vi "PRIME Gen Filenames and Log.vi"(9 "Observation":T1={"Priority"=0, "ID"="", "Observer"="", "Obj Name"="", "Obj Type"="", "RA and DEC String"={"RA"="HH:MM:SS.nnn", "DEC"="DEG:arcmin:arcsec.nn"}, "Filters"=[], "Integration Time"=0.0, "Observation Status"=enum."Error", "Offsets"={"RA"=0.0, "DEC"=0.0, "ROT"=0.0}, "Images"=0, "Dither Options"={"Dither"=enum."None", "Dither Radius"=0.0, "Dither Points"=0, "Dither Phase"=0.0, "B Offset"={"RA"=0.0, "DEC"=0.0}}, "Comment 1"="", "Comment 2"=""}, 10 "Detector Config":T8={"Detector"=0, "Offsets"=[[0, 0, 0, 0, 0, 0, 0, 0, 0, 0, 0, 0, 0, 0, 0, 0, 0, 0, 0, 0, 0, 0, 0, 0, 0, 0, 0, 0, 0, 0, 0, 0]], "Detector Computer"={"Machine"="192.168.121.11", "Password"="rSL!nux23456", "FITS File Path"="", "Port"=44444, "Header Path"="", "Name"=""}, "FITS hdr template0"=path "", "FITS hdr template1"=path "", "FITS Data File Path"=path "", "FITS Detector Settings"={"Exp Time Short"=0.0, "# of Frames"=0.0, "Exp Time Long"=0.0, "# of Groups"=0.0, "Object Name"="", "Object"="", "Obs Type"="", "Image Type"="", "Observer"="", "Observer Affiliation"=""}, "Sim Folder"=path "", "Integration Mode"=enum."Ramp", "Integration Time"=0.0, "Frame Int Time"=0.0} {"Offsets" format="%04x"; "Detector" items=["0", "1", "2"]}, 11 "Raw Files":T7) -> (0 "Exp Count out":i32, 1 "Source Files":path[](array[path]), 2 "Filenames":string[](array[string]), 3 "Table":string[](array[string]))   [LabVIEW 2024, in "PRIME Detector.lvclass"]
uses:
  PRIME Detector.lvclass
  RIMAS Detector Config.ctl
  RIMAS Detector Server Config.ctl
  RIMAS Observation Config.ctl
  Detector enum Detector Integration Mode.ctl
  Detector cluster Files.ctl
  typedefs/CC cluster Observation.ctl
  Observation Queue/CC enum Observation Status.ctl
  Telescope/CC cluster Telescope Offsets.ctl
  typedefs/CC cluster Observation Dither Options.ctl
  typedefs/CC enum Dither Selection.ctl
  typedefs/CC cluster RA and DEC.ctl
  PRIME Detector cluster Status.ctl
  FITS/PRIME cluster File Counter.ctl
  Logging/CC enum Current Values Action.ctl
  hk-channel-class/hk-channel-class/HK Table/HK Table.lvclass
  Detector Class.lvclass
panel:
  # "sec"
  # "sec"
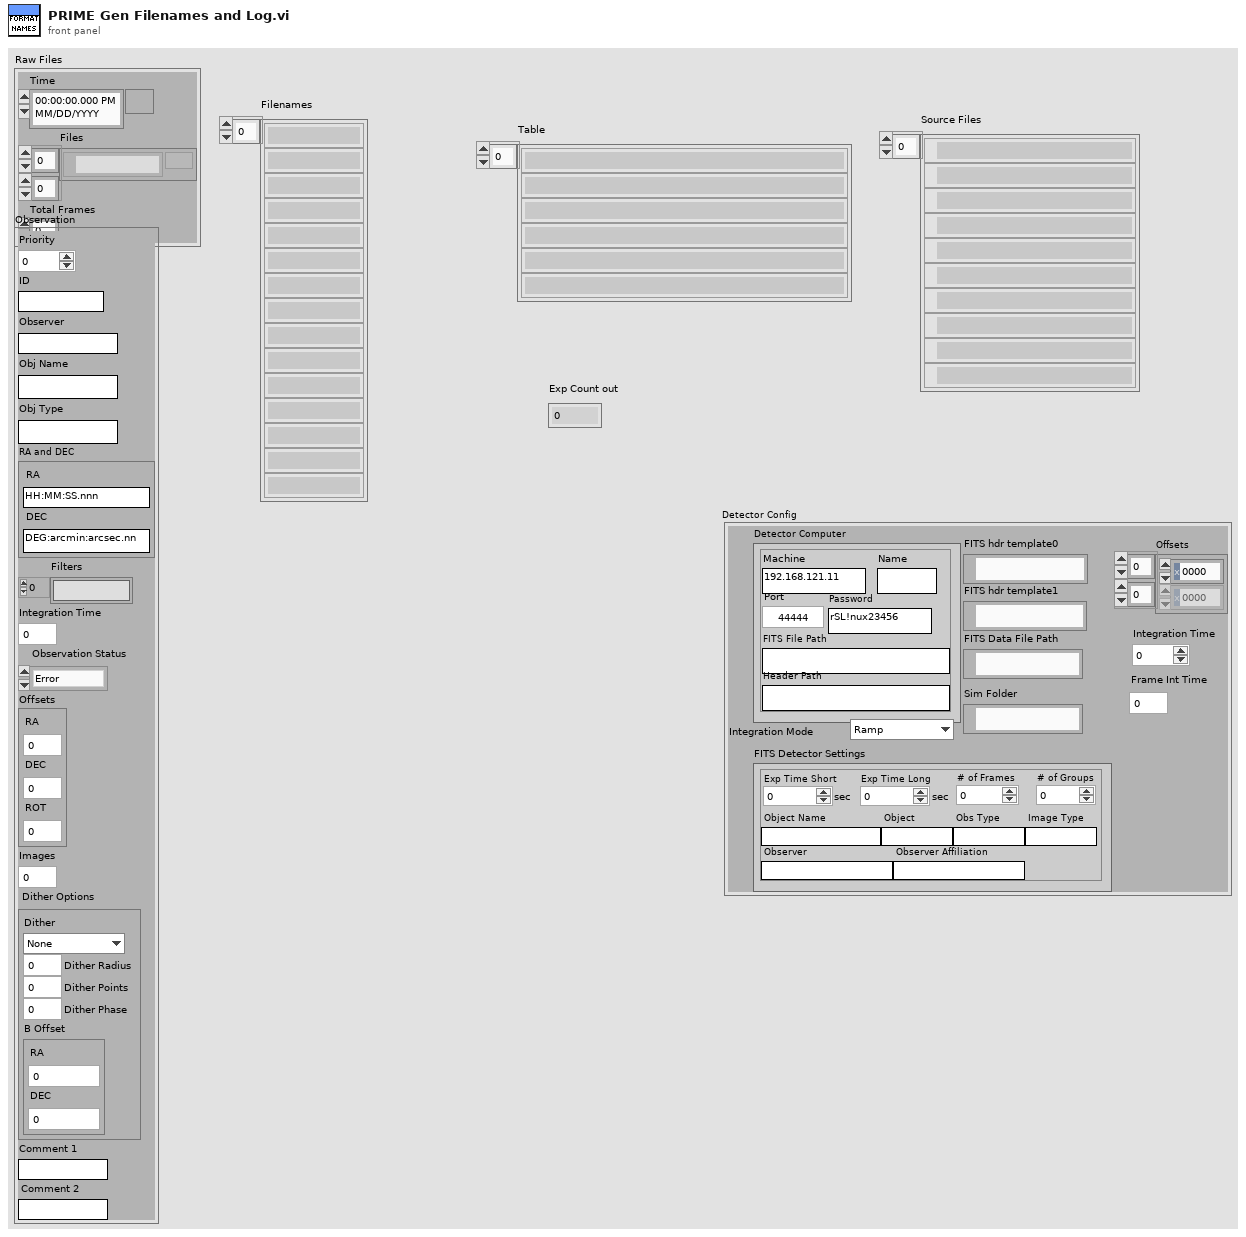
[diagram p1: front panel]
types:
  T1 = typedef "CC cluster Observation.ctl" = cluster{"Priority":i32, "ID":string, "Observer":string, "Obj Name":string, "Obj Type":string, "RA and DEC String":cluster{"RA":string, "DEC":string}, "Filters":string[], "Integration Time":dbl, "Observation Status":T2, "Offsets":T3, "Images":i32, "Dither Options":T4, "Comment 1":string, "Comment 2":string}
  T2 = typedef "CC enum Observation Status.ctl" = enum16{"Ready", "Running", "Done", "Error"}
  T3 = typedef "CC cluster Telescope Offsets.ctl" = cluster{"RA":dbl, "DEC":dbl, "ROT":dbl}
  T4 = typedef "CC cluster Observation Dither Options.ctl" = cluster{"Dither":T5, "Dither Radius":dbl, "Dither Points":i32, "Dither Phase":dbl, "B Offset":T6}
  T5 = typedef "CC enum Dither Selection.ctl" = enum16{"None", "Circle", "Random", "ABBA"}
  T6 = typedef "CC cluster RA and DEC.ctl" = cluster{"RA":dbl, "DEC":dbl}
  T7 = typedef "Detector Class.lvclass/Detector cluster Files.ctl" = cluster{"Time":timestamp, "Files":path[][], "Total Frames":i32}
  T8 = typedef "RIMAS Detector Config.ctl" = cluster{"Detector":u16, "Offsets":u16[][], "Detector Computer":T9, "FITS hdr template0":path, "FITS hdr template1":path, "FITS Data File Path":path, "FITS Detector Settings":T10, "Sim Folder":path, "Integration Mode":T11, "Integration Time":dbl, "Frame Int Time":dbl}
  T9 = typedef "RIMAS Detector Server Config.ctl" = cluster{"Machine":string, "Password":string, "FITS File Path":string, "Port":u16, "Header Path":string, "Name":string}
  T10 = typedef "RIMAS Observation Config.ctl" = cluster{"Exp Time Short":dbl, "# of Frames":dbl, "Exp Time Long":dbl, "# of Groups":dbl, "Object Name":string, "Object":string, "Obs Type":string, "Image Type":string, "Observer":string, "Observer Affiliation":string}
  T11 = typedef "Detector enum Detector Integration Mode.ctl" = enum16{"Ramp", "CDS", "FOWLER2", "FOWLER4", "FOWLER8", "FOWLER16", "Raw"}
  T12 = typedef "CC enum Current Values Action.ctl" = enum16{"Init", "Write Item", "Write Array", "Read Item", "Read Array", "Read All", "Add Channels", "New File", "Add Message", "Get Current Values", "Close"}
  T13 = typedef "PRIME cluster File Counter.ctl" = cluster{"File Count":i32}
  T14 = typedef "PRIME Detector cluster Status.ctl" = cluster{"Cmd Start Time":timestamp, "Command":string, "Complete?":bool, "Cmd Complete Time":timestamp, "Exp Time Remaining":dbl, "Total Frames":i32, "Exp Frames":cluster{"CAMERA0":string[], "CAMERA1":string[], "CAMERA2":string[], "CAMERA3":string[]}, "Intermediate Frames":cluster{"CAMERA0":string[], "CAMERA1":string[], "CAMERA2":string[], "CAMERA3":string[]}, "Final Reduced Frame":cluster{"CAMERA0":string, "CAMERA1":string, "CAMERA2":string, "CAMERA3":string}}
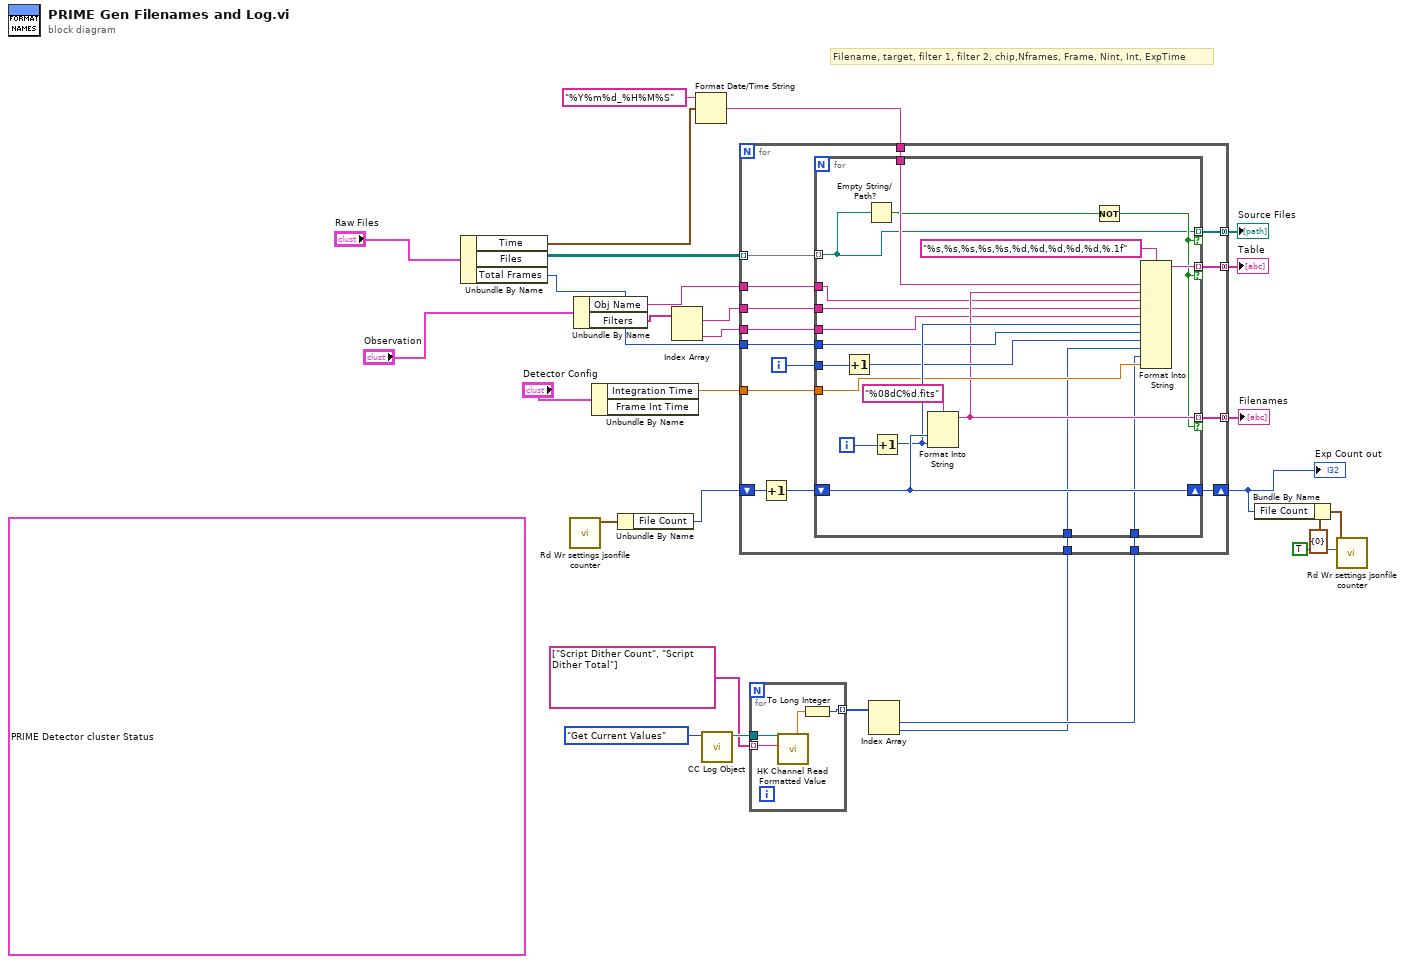
[diagram p0: block diagram]
diagram:
  (unwired) T14 {"Cmd Start Time"=timestamp(3729599083.065959 s since 1904-01-01), "Command"="START", "Complete?"=TRUE, "Cmd Complete Time"=timestamp(3729599162.21691 s since 1904-01-01), "Exp Time Remaining"=0.0, "Total Frames"=8, "Exp Frames"={"CAMERA0"=["C:\\Users\\gsfcprime\\PycharmProjects\\asdetector\\output\\raw\\20220308\\prime.0000.C0\\prime.0000.C0.000000.fits", "C:\\Users\\gsfcprime\\PycharmProjects\\asdetector\\output\\raw\\20220308\\prime.0000.C0\\prime.0000.C0.000001.fits", "C:\\Users\\gsfcprime\\PycharmProjects\\asdetector\\output\\raw\\20220308\\prime.0000.C0\\prime.0000.C0.000002.fits", "C:\\Users\\gsfcprime\\PycharmProjects\\asdetector\\output\\raw\\20220308\\prime.0000.C0\\prime.0000.C0.000003.fits", "C:\\Users\\gsfcprime\\PycharmProjects\\asdetector\\output\\raw\\20220308\\prime.0000.C0\\prime.0000.C0.000004.fits", "C:\\Users\\gsfcprime\\PycharmProjects\\asdetector\\output\\raw\\20220308\\prime.0000.C0\\prime.0000.C0.000005.fits", "C:\\Users\\gsfcprime\\PycharmProjects\\asdetector\\output\\raw\\20220308\\prime.0000.C0\\prime.0000.C0.000006.fits", "C:\\Users\\gsfcprime\\PycharmProjects\\asdetector\\output\\raw\\20220308\\prime.0000.C0\\prime.0000.C0.000007.fits"], "CAMERA1"=["C:\\Users\\gsfcprime\\PycharmProjects\\asdetector\\output\\raw\\20220308\\prime.0000.C1\\prime.0000.C1.000000.fits", "C:\\Users\\gsfcprime\\PycharmProjects\\asdetector\\output\\raw\\20220308\\prime.0000.C1\\prime.0000.C1.000001.fits", "C:\\Users\\gsfcprime\\PycharmProjects\\asdetector\\output\\raw\\20220308\\prime.0000.C1\\prime.0000.C1.000002.fits", "C:\\Users\\gsfcprime\\PycharmProjects\\asdetector\\output\\raw\\20220308\\prime.0000.C1\\prime.0000.C1.000003.fits", "C:\\Users\\gsfcprime\\PycharmProjects\\asdetector\\output\\raw\\20220308\\prime.0000.C1\\prime.0000.C1.000004.fits", "C:\\Users\\gsfcprime\\PycharmProjects\\asdetector\\output\\raw\\20220308\\prime.0000.C1\\prime.0000.C1.000005.fits", "C:\\Users\\gsfcprime\\PycharmProjects\\asdetector\\output\\raw\\20220308\\prime.0000.C1\\prime.0000.C1.000006.fits", "C:\\Users\\gsfcprime\\PycharmProjects\\asdetector\\output\\raw\\20220308\\prime.0000.C1\\prime.0000.C1.000007.fits"], "CAMERA2"=["C:\\Users\\gsfcprime\\PycharmProjects\\asdetector\\output\\raw\\20220308\\prime.0000.C2\\prime.0000.C2.000000.fits", "C:\\Users\\gsfcprime\\PycharmProjects\\asdetector\\output\\raw\\20220308\\prime.0000.C2\\prime.0000.C2.000001.fits", "C:\\Users\\gsfcprime\\PycharmProjects\\asdetector\\output\\raw\\20220308\\prime.0000.C2\\prime.0000.C2.000002.fits", "C:\\Users\\gsfcprime\\PycharmProjects\\asdetector\\output\\raw\\20220308\\prime.0000.C2\\prime.0000.C2.000003.fits", "C:\\Users\\gsfcprime\\PycharmProjects\\asdetector\\output\\raw\\20220308\\prime.0000.C2\\prime.0000.C2.000004.fits", "C:\\Users\\gsfcprime\\PycharmProjects\\asdetector\\output\\raw\\20220308\\prime.0000.C2\\prime.0000.C2.000005.fits", "C:\\Users\\gsfcprime\\PycharmProjects\\asdetector\\output\\raw\\20220308\\prime.0000.C2\\prime.0000.C2.000006.fits", "C:\\Users\\gsfcprime\\PycharmProjects\\asdetector\\output\\raw\\20220308\\prime.0000.C2\\prime.0000.C2.000007.fits"], "CAMERA3"=["C:\\Users\\gsfcprime\\PycharmProjects\\asdetector\\output\\raw\\20220308\\prime.0000.C3\\prime.0000.C3.000000.fits", "C:\\Users\\gsfcprime\\PycharmProjects\\asdetector\\output\\raw\\20220308\\prime.0000.C3\\prime.0000.C3.000001.fits", "C:\\Users\\gsfcprime\\PycharmProjects\\asdetector\\output\\raw\\20220308\\prime.0000.C3\\prime.0000.C3.000002.fits", "C:\\Users\\gsfcprime\\PycharmProjects\\asdetector\\output\\raw\\20220308\\prime.0000.C3\\prime.0000.C3.000003.fits", "C:\\Users\\gsfcprime\\PycharmProjects\\asdetector\\output\\raw\\20220308\\prime.0000.C3\\prime.0000.C3.000004.fits", "C:\\Users\\gsfcprime\\PycharmProjects\\asdetector\\output\\raw\\20220308\\prime.0000.C3\\prime.0000.C3.000005.fits", "C:\\Users\\gsfcprime\\PycharmProjects\\asdetector\\output\\raw\\20220308\\prime.0000.C3\\prime.0000.C3.000006.fits", "C:\\Users\\gsfcprime\\PycharmProjects\\asdetector\\output\\raw\\20220308\\prime.0000.C3\\prime.0000.C3.000007.fits"]}, "Intermediate Frames"={"CAMERA0"=["C:\\Users\\gsfcprime\\PycharmProjects\\asdetector\\output\\res\\20220308\\prime.0000.C0\\prime.0000.C0.000000.fits", "C:\\Users\\gsfcprime\\PycharmProjects\\asdetector\\output\\res\\20220308\\prime.0000.C0\\prime.0000.C0.000001.fits", "C:\\Users\\gsfcprime\\PycharmProjects\\asdetector\\output\\res\\20220308\\prime.0000.C0\\prime.0000.C0.000002.fits", "C:\\Users\\gsfcprime\\PycharmProjects\\asdetector\\output\\res\\20220308\\prime.0000.C0\\prime.0000.C0.000003.fits", "C:\\Users\\gsfcprime\\PycharmProjects\\asdetector\\output\\res\\20220308\\prime.0000.C0\\prime.0000.C0.000004.fits", "C:\\Users\\gsfcprime\\PycharmProjects\\asdetector\\output\\res\\20220308\\prime.0000.C0\\prime.0000.C0.000005.fits", "C:\\Users\\gsfcprime\\PycharmProjects\\asdetector\\output\\res\\20220308\\prime.0000.C0\\prime.0000.C0.000006.fits", "C:\\Users\\gsfcprime\\PycharmProjects\\asdetector\\output\\res\\20220308\\prime.0000.C0\\prime.0000.C0.000007.fits"], "CAMERA1"=["C:\\Users\\gsfcprime\\PycharmProjects\\asdetector\\output\\res\\20220308\\prime.0000.C1\\prime.0000.C1.000000.fits", "C:\\Users\\gsfcprime\\PycharmProjects\\asdetector\\output\\res\\20220308\\prime.0000.C1\\prime.0000.C1.000001.fits", "C:\\Users\\gsfcprime\\PycharmProjects\\asdetector\\output\\res\\20220308\\prime.0000.C1\\prime.0000.C1.000002.fits", "C:\\Users\\gsfcprime\\PycharmProjects\\asdetector\\output\\res\\20220308\\prime.0000.C1\\prime.0000.C1.000003.fits", "C:\\Users\\gsfcprime\\PycharmProjects\\asdetector\\output\\res\\20220308\\prime.0000.C1\\prime.0000.C1.000004.fits", "C:\\Users\\gsfcprime\\PycharmProjects\\asdetector\\output\\res\\20220308\\prime.0000.C1\\prime.0000.C1.000005.fits", "C:\\Users\\gsfcprime\\PycharmProjects\\asdetector\\output\\res\\20220308\\prime.0000.C1\\prime.0000.C1.000006.fits", "C:\\Users\\gsfcprime\\PycharmProjects\\asdetector\\output\\res\\20220308\\prime.0000.C1\\prime.0000.C1.000007.fits"], "CAMERA2"=["C:\\Users\\gsfcprime\\PycharmProjects\\asdetector\\output\\res\\20220308\\prime.0000.C2\\prime.0000.C2.000000.fits", "C:\\Users\\gsfcprime\\PycharmProjects\\asdetector\\output\\res\\20220308\\prime.0000.C2\\prime.0000.C2.000001.fits", "C:\\Users\\gsfcprime\\PycharmProjects\\asdetector\\output\\res\\20220308\\prime.0000.C2\\prime.0000.C2.000002.fits", "C:\\Users\\gsfcprime\\PycharmProjects\\asdetector\\output\\res\\20220308\\prime.0000.C2\\prime.0000.C2.000003.fits", "C:\\Users\\gsfcprime\\PycharmProjects\\asdetector\\output\\res\\20220308\\prime.0000.C2\\prime.0000.C2.000004.fits", "C:\\Users\\gsfcprime\\PycharmProjects\\asdetector\\output\\res\\20220308\\prime.0000.C2\\prime.0000.C2.000005.fits", "C:\\Users\\gsfcprime\\PycharmProjects\\asdetector\\output\\res\\20220308\\prime.0000.C2\\prime.0000.C2.000006.fits", "C:\\Users\\gsfcprime\\PycharmProjects\\asdetector\\output\\res\\20220308\\prime.0000.C2\\prime.0000.C2.000007.fits"], "CAMERA3"=["C:\\Users\\gsfcprime\\PycharmProjects\\asdetector\\output\\res\\20220308\\prime.0000.C3\\prime.0000.C3.000000.fits", "C:\\Users\\gsfcprime\\PycharmProjects\\asdetector\\output\\res\\20220308\\prime.0000.C3\\prime.0000.C3.000001.fits", "C:\\Users\\gsfcprime\\PycharmProjects\\asdetector\\output\\res\\20220308\\prime.0000.C3\\prime.0000.C3.000002.fits", "C:\\Users\\gsfcprime\\PycharmProjects\\asdetector\\output\\res\\20220308\\prime.0000.C3\\prime.0000.C3.000003.fits", "C:\\Users\\gsfcprime\\PycharmProjects\\asdetector\\output\\res\\20220308\\prime.0000.C3\\prime.0000.C3.000004.fits", "C:\\Users\\gsfcprime\\PycharmProjects\\asdetector\\output\\res\\20220308\\prime.0000.C3\\prime.0000.C3.000005.fits", "C:\\Users\\gsfcprime\\PycharmProjects\\asdetector\\output\\res\\20220308\\prime.0000.C3\\prime.0000.C3.000006.fits", "C:\\Users\\gsfcprime\\PycharmProjects\\asdetector\\output\\res\\20220308\\prime.0000.C3\\prime.0000.C3.000007.fits"]}, "Final Reduced Frame"={"CAMERA0"="C:\\Users\\gsfcprime\\PycharmProjects\\asdetector\\output\\reduced\\20220308\\prime.0000.C0.fits", "CAMERA1"="C:\\Users\\gsfcprime\\PycharmProjects\\asdetector\\output\\reduced\\20220308\\prime.0000.C1.fits", "CAMERA2"="C:\\Users\\gsfcprime\\PycharmProjects\\asdetector\\output\\reduced\\20220308\\prime.0000.C2.fits", "CAMERA3"="C:\\Users\\gsfcprime\\PycharmProjects\\asdetector\\output\\reduced\\20220308\\prime.0000.C3.fits"}} ("prime detector status")
  # "Filename, target, filter 1, filter 2, chip,Nframes, Frame, Nint, Int, ExpTime"
  n1 = Unbundle By Name("Raw Files") -> ("Time"=w8:timestamp, "Files"=w7:path[][], "Total Frames"=w6:i32)
  n2 = call "Rd Wr settings jsonfile counter.vi"() -> ("FileCounter"=w21:T13)  [unwired: 10 in, 1 out]
  n3 = Unbundle By Name("Observation") -> ("Obj Name"=w3:string, "Filters"=w4:string[])
  n4 = Unbundle By Name("Detector Config") -> ("Integration Time"=w26:dbl)  [unwired: 1 out]
  n5 = Unbundle By Name(w21) -> ("File Count"=w20:i32)
  n6 = Index Array(array=w4) -> (element #1=w2:string, element #2=w1:string)  [unwired: 2 in]
  n7 = Format Date/Time String(time format string (%c)="%Y%m%d_%H%M%S", seconds (now)=w8) -> (date/time string=w22:string)  [unwired: 1 in]
  n8 = call "CC Log Object.vi"("Action"=CC_enum_Current_Values_Action."Get Current Values") -> ("HK Channel out"=w14:refnum<class "HK Table.lvclass">)  [unwired: 8 in, 2 out]
  n9 = for {
    tunnel: w14 -> [w32]
    tunnel: string[] ["Script Dither Count", "Script Dither Total"] -> [w31] mode=indexing
    tunnel: [w29] -> w12 mode=indexing
    n10 = call-dynamic "HK Channel Read Formatted Value.vi"("Name"=w31, "HK Table.lvclass"=w32) -> ("Value"=w30:dbl)  [unwired: 2 in, 7 out]
    n11 = To Long Integer(number=w30) -> (32bit integer=w29:i32)
  }
  n12 = Index Array(array=w12) -> (element #1=w11:i32, element #2=w10:i32)  [unwired: 2 in]
  n13 = for {
    shift-right: [w48] -> w18
    shift-left: w20 -> [w47]
    tunnel: w7 -> [w46] mode=indexing
    tunnel: [w44] -> w28 mode=concatenating
    tunnel: w6 -> [w43]
    tunnel: w11 -> [w41]
    tunnel: w26 -> [w40]
    tunnel: [w39] -> w25 mode=concatenating
    tunnel: [w38] -> w24 mode=concatenating
    tunnel: w22 -> [w37]
    tunnel: w10 -> [w36]
    tunnel: w1 -> [w35]
    tunnel: w2 -> [w34]
    tunnel: w3 -> [w33]
    i -> [w42]
    n14 = Increment(x=w47) -> (x+1=w45:i32)
    n15 = for {
      shift-right: [w67] -> w48
      shift-left: w45 -> [w67]
      tunnel: w46 -> [w52] mode=indexing
      tunnel: [w58] -> w44 mode=indexing if=w56
      tunnel: w43 -> [w63]
      tunnel: w42 -> [w62]
      tunnel: w41 -> [w54]
      tunnel: w40 -> [w60]
      tunnel: [w59] -> w39 mode=indexing if=w56
      tunnel: [w52] -> w38 mode=indexing if=w56
      tunnel: w37 -> [w57]
      tunnel: w36 -> [w53]
      tunnel: w35 -> [w51]
      tunnel: w34 -> [w50]
      tunnel: w33 -> [w49]
      i -> [w66]
      n16 = Increment(x=w62) -> (x+1=w61:i32)
      n17 = Empty String/Path?(string/path=w52) -> (empty?=w55:bool)
      n18 = Increment(x=w66) -> (x+1=w64:i32)
      n19 = Format Into String(format string="%08dC%d.fits", w67, w64) -> (resulting string=w58:string)  [unwired: 2 in, 1 out]
      n20 = Not(x=w55) -> (.not. x?=w56:bool)
      n21 = Format Into String(format string="%s,%s,%s,%s,%s,%d,%d,%d,%d,%d,%.1f", w57, w58, w49, w50, w51, w64, w63, w61, w53, w54, w60) -> (resulting string=w59:string)  [unwired: 2 in, 1 out]
    }
  }
  "Filenames" <- w28
  "Table" <- w25
  "Exp Count out" <- w18
  "Source Files" <- w24
  n22 = Bundle By Name(cluster=T13 {"File Count"=0}, "File Count"=w18) -> (w17:T13)
  n23 = call "Rd Wr settings jsonfile counter.vi"("Write? (F:Read)"=TRUE, "FileCounter"=w17) -> ()  [unwired: 8 in, 2 out]
